vi "MartinsDCtemp.vi"() -> ()   [LabVIEW 2011]
uses:
  Sub VIs/Trap cluster.ctl
  <vilib>/Utility/inputDevices.llb/closeKeyboard.vi
  <vilib>/Utility/inputDevices.llb/keyboardAcquire.vi
  <vilib>/Utility/file.llb/Write To Spreadsheet File (DBL).vi
  <vilib>/vision/driver/NI_Vision_Acquisition_Software.lvlib
panel:
  in  "e_desired":sgl=0.5
  in  "Apply Corrections":bool
  in  "View Licence":bool
  in  "ok":bool caption="Mark the center of \nthe spot using the \nzoom and the point\ntool, then click this \nbutton"
  in  "Stop program":bool
  in  "Updating trap cluster":bool
  out "Camera enabled":bool
  out "SLM enabled":bool
  in  "Run calibration":bool
  in  "Hologram generation":cluster{"Method":i32, "Iterations":i32}={"Method"=0, "Iterations"=10} {"Method" items=["Lenses & Gratings (3D)", " Gerchberg-Saxton (3D)", "Gerchberg-Saxton FFT (2D)"]}
  in  "Display hologram\nand computed \nimage plane":bool=TRUE
  in  "ROI":T1={"Global Rectangle"=[309, 286, 371, 364], "Contours"=[{"Contour Type"=0, "ROI Type"=1, "Points"=[370, 286]}, {"Contour Type"=0, "ROI Type"=1, "Points"=[351, 363]}, {"Contour Type"=0, "ROI Type"=1, "Points"=[309, 315]}]}
  out "Image":T2(plugin-control)
  in  "Filename":string="test"
  out "appended path":path
  in  "File Path":path=path "C:/Users/Martin/Dropbox/GU/CUDA/GenerateHologramCUDA/LabVIEW/MartinDC/Measurements"
  in  "Save images":bool
  in  "Show image":bool=TRUE
  in  "ROI size":dbl=2.0 min=2.0 step=2.0
  in  "#images":i32=10
  in  "Tab Control":enum32{"Normal", "Grid"}(tab)=enum."Grid"
  in  "Z":dbl[](array[numeric])=[0.0, 0.0, 0.0]
  in  "I":dbl[](array[numeric])=[10.0, 10.0, 10.0]
  out "#":i32[](array[numeric])=[0, 1, 2]
  in  "G":bool[](array[boolean])=[FALSE, FALSE, FALSE]
  in  "Spots y":i32=3
  in  "Grid spacing":i32=32
  in  "Spots x":i32=3
  out "Calculated image plane":dbl[][](graph)
  out "Current trap pos":T3
  out "NI Vision error":errorcluster
  out "CUDA/SLM error":errorcluster
  in  "Cancel calibration":bool
  in  "Skip step if \ntimed out":bool
  in  "Display path":bool=TRUE
  out "Average step time (ms)":dbl
  in  "Step time \n(ms)":u32=10
  in  "Pause":bool
  in  "cancel path":bool
  out "Step skipped":bool
  in  "Path controls":T4={"follow path"=FALSE, "Step length"=1.0, "Arrive \nsimultaneously"=TRUE, "Synchronize traps"=FALSE, "Add current \npositions to path"=FALSE}
  in  "Create path":bool
  in  "Positioning  mode":enum16{"Normal", "Group", "Grid"}(ring)=enum."Grid"
  in  "Move \nHandle":bool
  out "Displayed Hologram":u8[][](graph)
  in  "Coordinate mapping \n(IMAQ to SLM)":T5={"sX"=-256.0, "sY"=-256.0, "sZ"=0.0, "cX"=0.5, "cY"=0.5, "cZ"=1.0}
  in  "Switch X/Y":bool
  # "Martin\nPersson 2011"
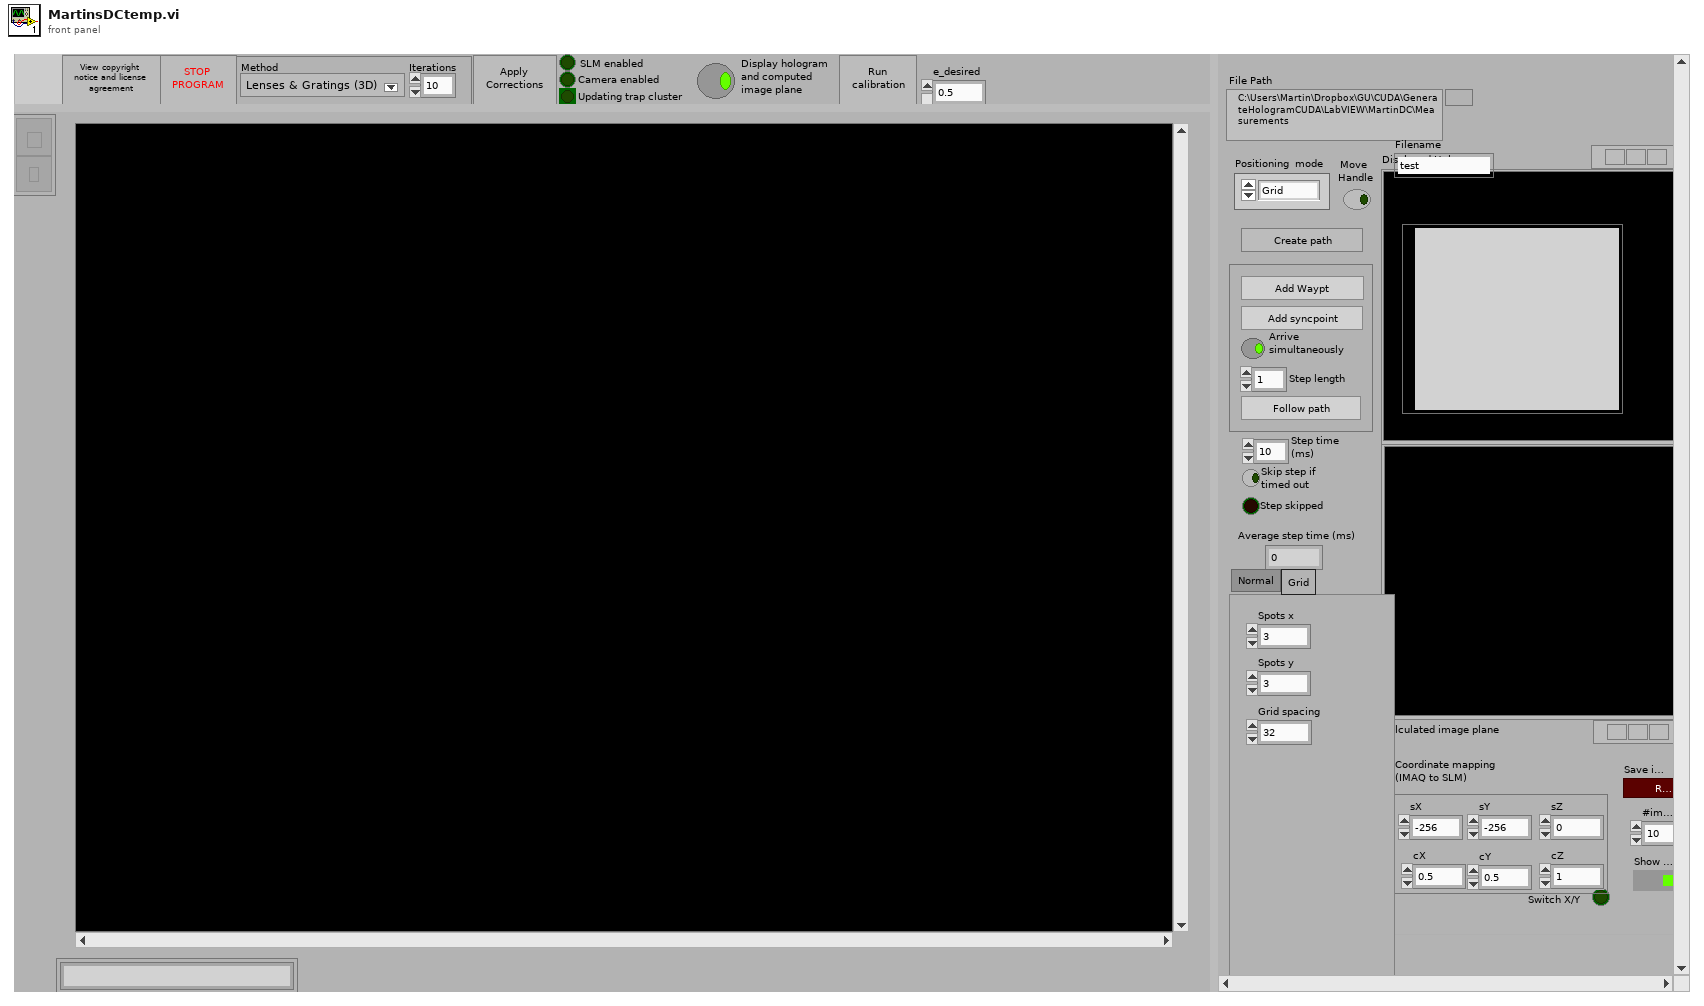
[diagram p1: front panel]
types:
  T1 = cluster{"Global Rectangle":i32[], "Contours":cluster{"Contour Type":u32, "ROI Type":u32, "Points":i32[]}[]}
  T2 = typedef "IMAQ Image.ctl" = refnum<image>
  T3 = typedef "Trap cluster.ctl" = cluster{"X (IMAQ)":dbl[], "Y (IMAQ)":dbl[], "Z":dbl[], "Amplitudes":dbl[], "Trap number":i32[], "ROI number":i32[], "Number of traps":i32, "Group":bool[]}
  T4 = cluster{"follow path":bool, "Step length":dbl, "Arrive \nsimultaneously":bool, "Synchronize traps":bool, "Add current \npositions to path":bool}
  T5 = cluster{"sX":dbl, "sY":dbl, "sZ":dbl, "cX":dbl, "cY":dbl, "cZ":dbl}
  T6 = cluster{"Centroid X":dbl[], "Centroid Y":dbl[], "Acquired Buffer Number":u32}
  T7 = typedef "IMAQdx.ctl" = refnum<k21>
  T8 = typedef "Image Type" = u32
  T9 = enum16{"0", "1", "2", "3", "4", "5", "6", "7", "8", "9", "A", "B", "C", "D", "E", "F", "G", "H", "I", "J", "K", "L", "M", "N", "O", "P", "Q", "R", "S", "T", "U", "V", "W", "X", "Y", "Z", "F1", "F2", "F3", "F4", "F5", "F6", "F7", "F8", "F9", "F10", "F11", "F12", "F13", "F14", "F15", "ADD", "BACK", "BACKSLASH", "CAPITAL", "COMMA", "DECIMAL", "DELETE", "DIVIDE", "DOWN", "END", "EQUALS", "ESCAPE", "GRAVE (`)", "HOME", "INSERT", "LBRACKET", "LCONTROL", "LEFT", "L ALT", "LSHIFT", "LWIN", "MINUS", "MULTIPLY", "NEXT", "NUMLOCK", "NUMPAD_0", "NUMPAD_1", "NUMPAD_2", "NUMPAD_3", "NUMPAD_4", "NUMPAD_5", "NUMPAD_6", "NUMPAD_7", "NUMPAD_8", "NUMPAD_9", "PAUSE", "PERIOD", "PRIOR (PG UP)", "RBRACKET", "RCONTROL", "RETURN", "RIGHT", "R ALT", "RSHIFT", "RWIN", "SCROLL", "SEMICOLON", "SLASH", "SPACE", "SUBTRACT", "TAB", "UP", "ENTER (num pad)", "' (quote)"}[]
  T10 = typedef "LVRectTypeDef.ctl" = cluster{"left":i16, "top":i16, "right":i16, "bottom":i16}
  T11 = cluster{"Contour Type":u32, "ROI Type":u32, "Points":i32[]}[]
  T12 = cluster{"Contour Type":u32, "ROI Type":u32, "Points":i32[]}
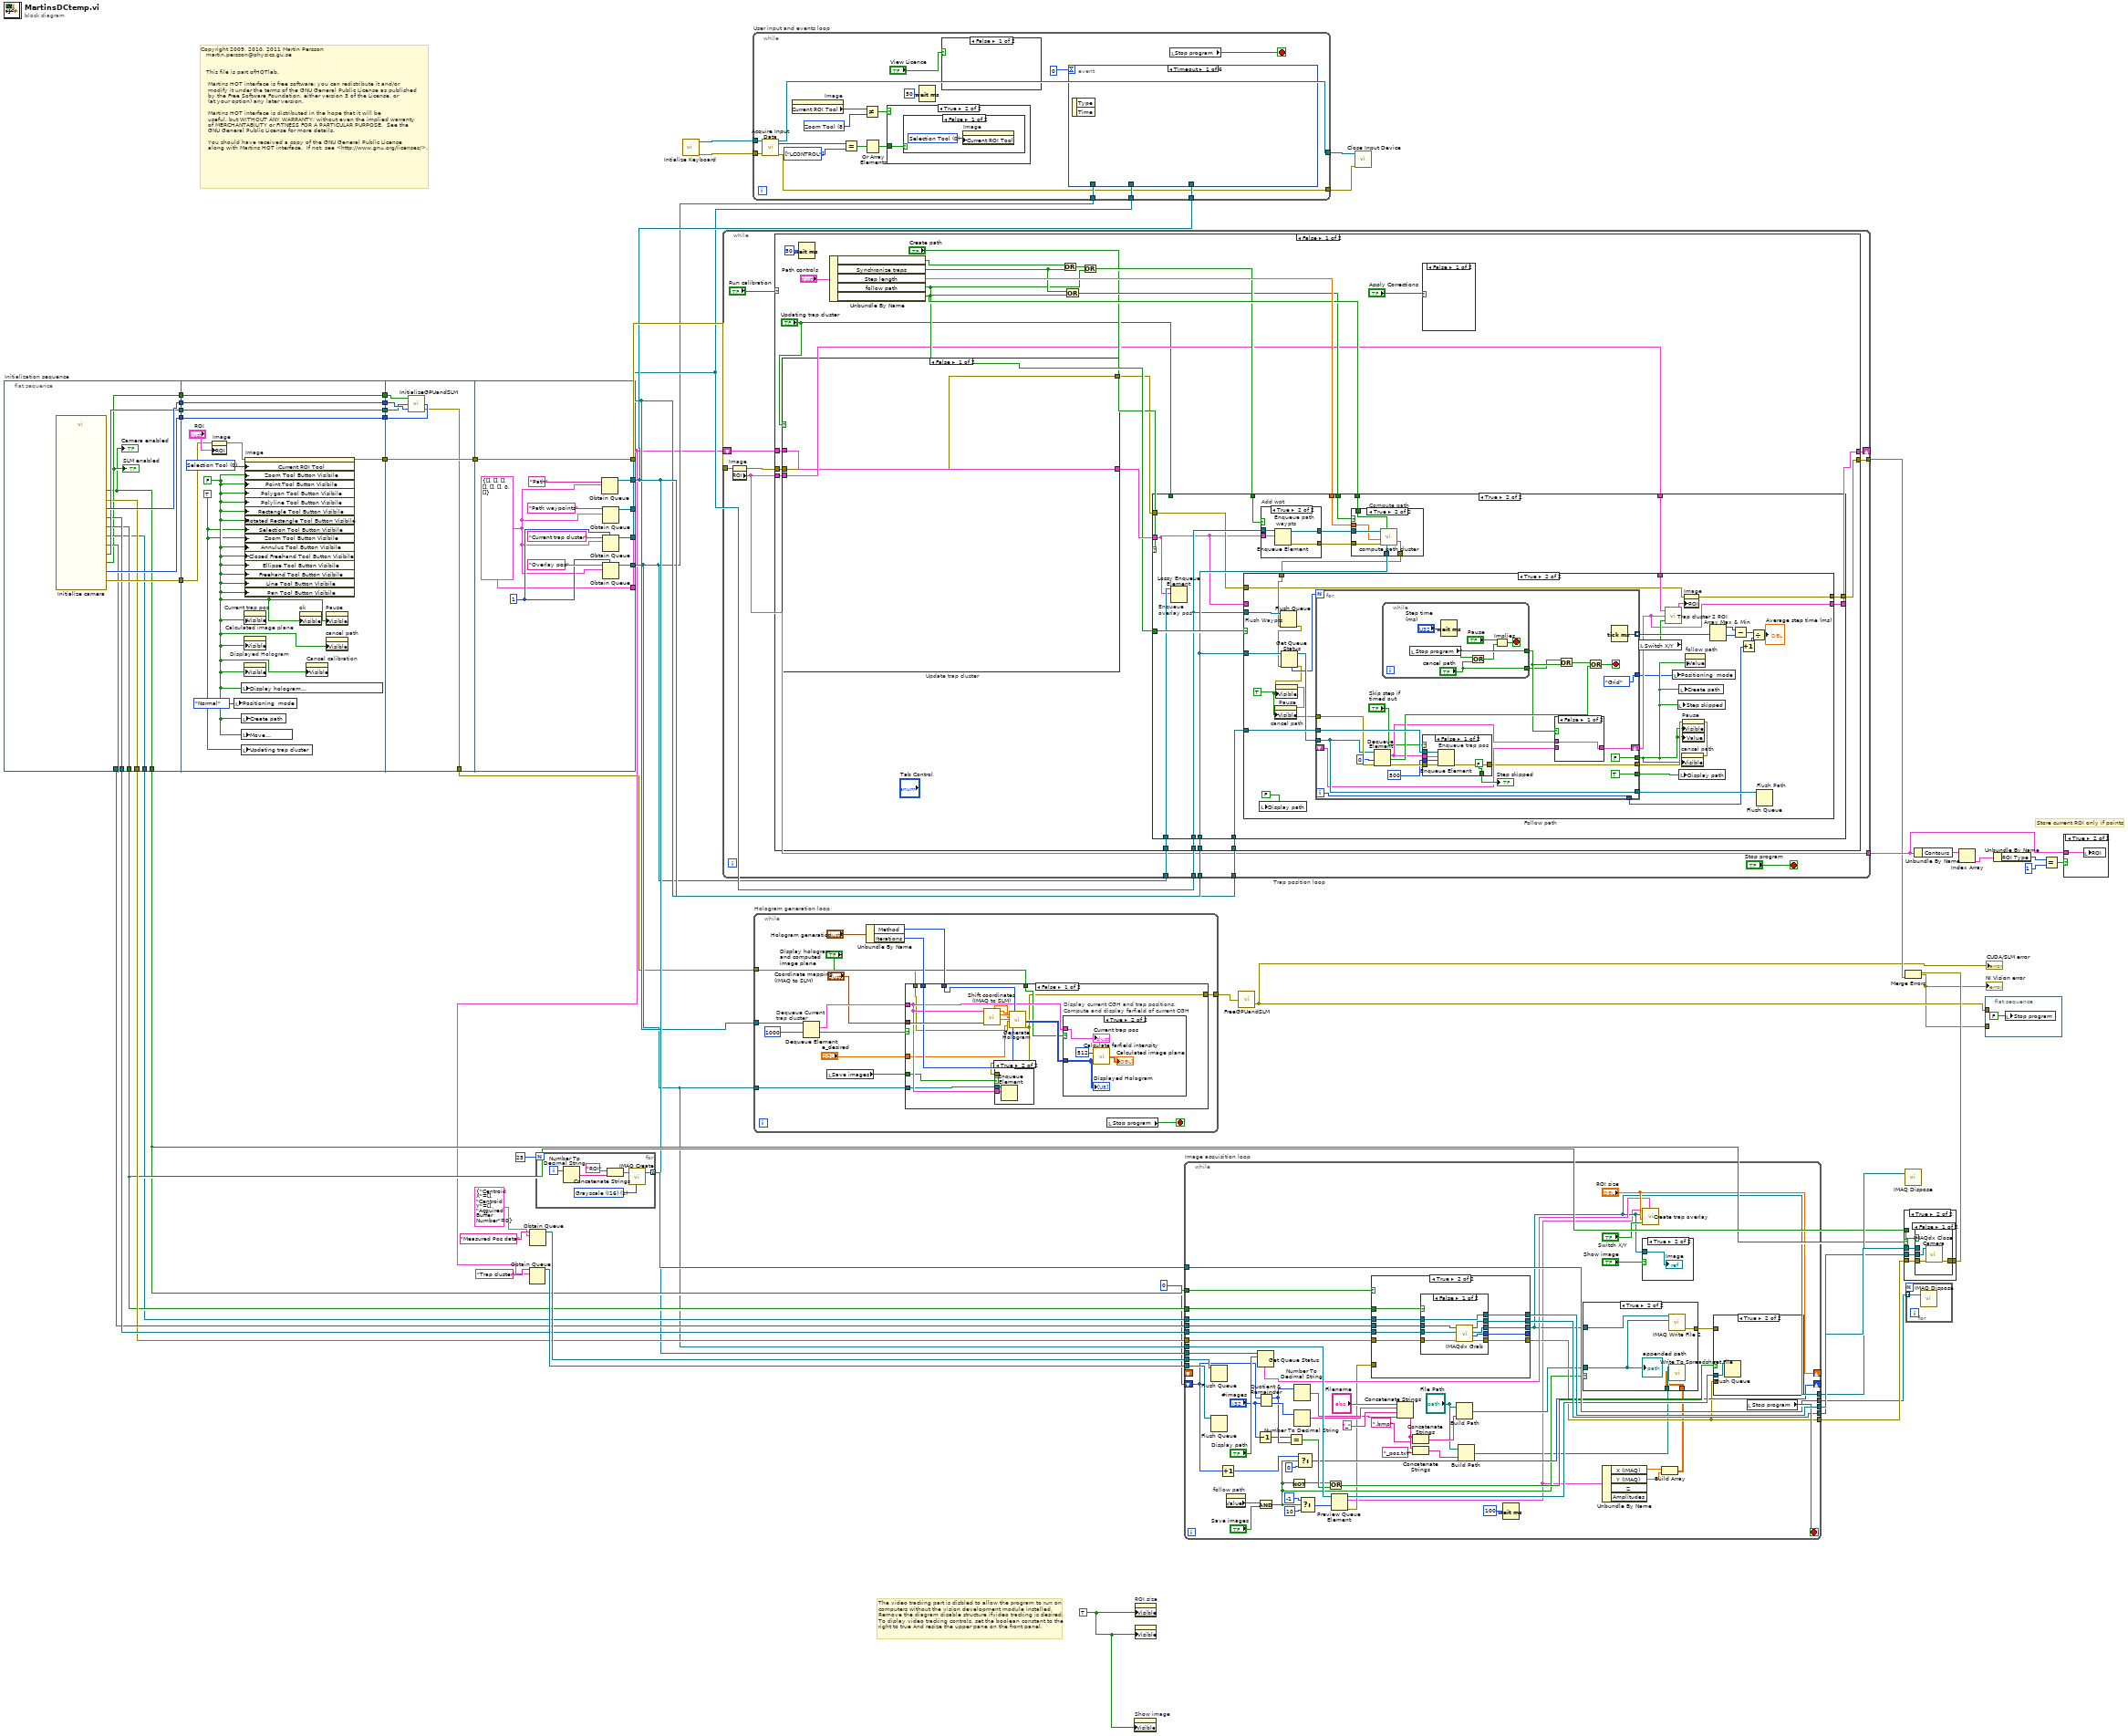
[diagram p0: block diagram]
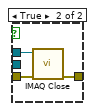
[diagram p3: hidden frame]
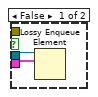
[diagram p4: hidden frame]
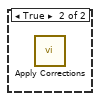
[diagram p7: hidden frame]
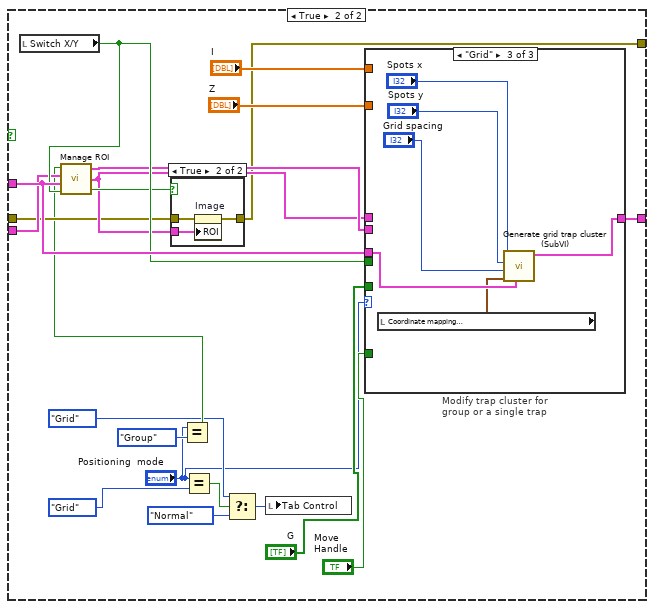
[diagram p8: hidden frame]
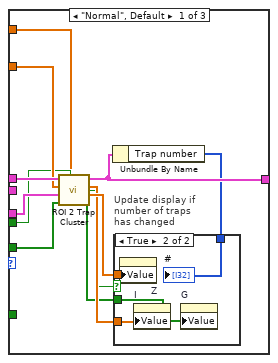
[diagram p10: hidden frame]
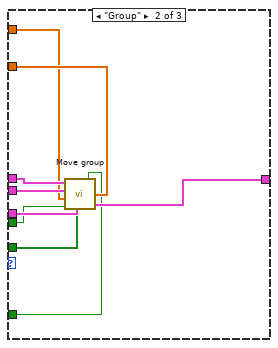
[diagram p12: hidden frame]
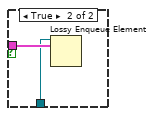
[diagram p14: hidden frame]
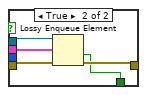
[diagram p16: hidden frame]
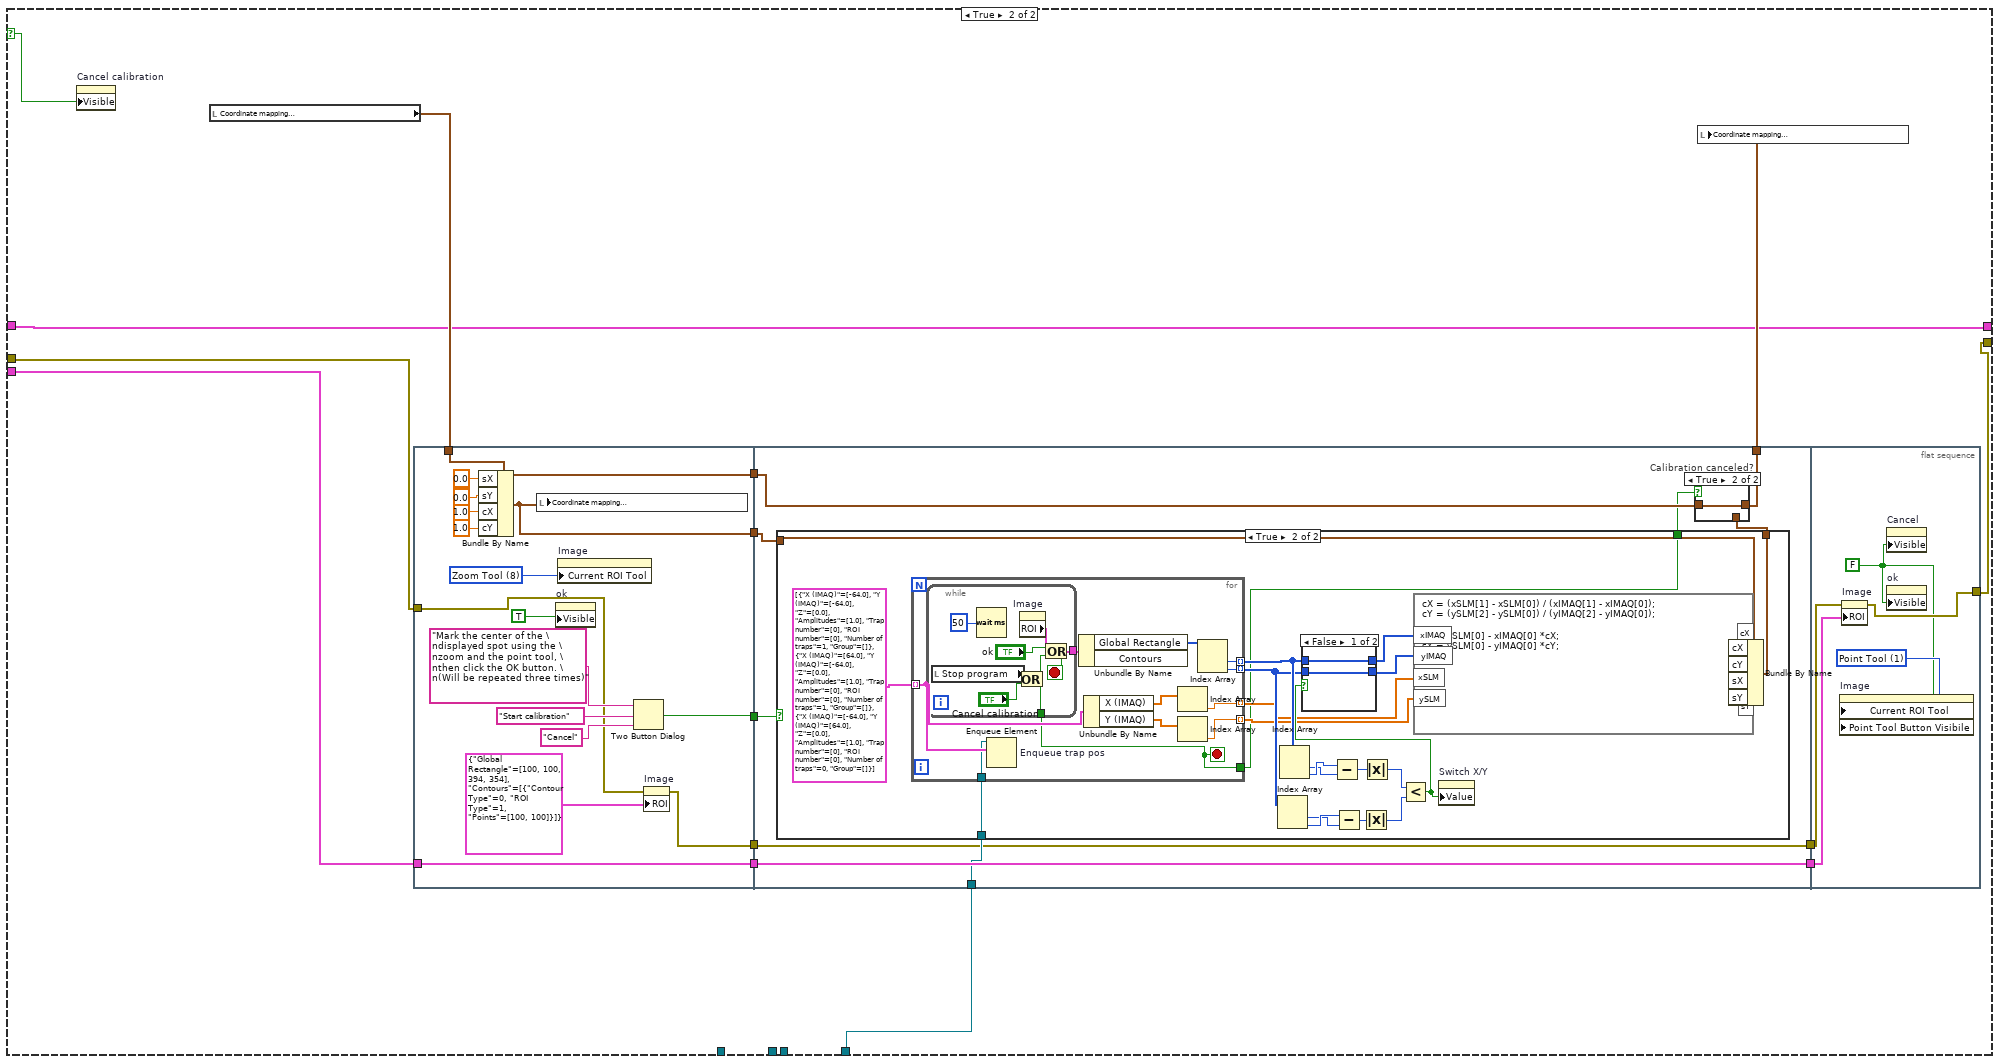
[diagram p20: hidden frame]
diagram:
  w40 = TRUE ("Visible")
  # "Copyright 2009, 2010, 2011 Martin Persson \n   martin.persson@physics.gu.se\n\n\n   This file is part ofHOTlab.\n\n    Martins HOT interface is free software: you can redistribute it and/or \n    modify it under the terms of the GNU General Public License as published \n    by the Free Software Foundation, either version 3 of the License, or\n    (at your option) any later version.\n\n    Martins HOT interface is distributed in the hope that it will be \n    useful, but WITHOUT ANY WARRANTY; without even the implied warranty\n    of MERCHANTABILITY or FITNESS FOR A PARTICULAR PURPOSE.  See the\n    GNU General Public License for more details.\n\n    You should have received a copy of the GNU General Public License\n    along with Martins HOT interface.  If not, see <http://www.gnu.org/licenses/>."
  # "Store current ROI only if points"
  # "The video tracking part is disbled to allow the program to run on\ncomputers without the vision development module installed. \nRemove the diagram disable structure ifvideo tracking is desired. \nTo diplay video tracking controls, set the boolean constant to the \nright to true And resize the upper pane on the front panel."
  n1 = flat-sequence "Initialization sequence" {
    tunnel: [w55] -> w25
    tunnel: [w64] -> w24
    tunnel: [w63] -> w23
    tunnel: [w62] -> w22
    tunnel: [w61] -> w21
    tunnel: [w60] -> w19
    tunnel: [w59] -> w18
    tunnel: [w58] -> w17
    tunnel: [w57] -> w16
    tunnel: [w56] -> w15
    tunnel: [w54] -> w14
    tunnel: w25 -> [w73]
    tunnel: w24 -> [w71]
    tunnel: w23 -> [w76]
    tunnel: w22 -> [w75]
    tunnel: w21 -> [w74]
    tunnel: [w73] -> w8
    tunnel: [w66] -> w7
    tunnel: [w76] -> w5
    tunnel: [w75] -> w4
    tunnel: [w74] -> w3
    tunnel: w8 -> [w79]
    tunnel: w7 -> [w82]
    tunnel: [w82] -> w6
    tunnel: w5 -> [w80]
    tunnel: w4 -> [w81]
    tunnel: w3 -> [w78]
    tunnel: [w77] -> w2
    tunnel: [w93] -> w20
    tunnel: w6 -> [w93]
    tunnel: [w91] -> w13
    tunnel: [w89] -> w12
    tunnel: [w87] -> w11
    tunnel: [w86] -> w10
    tunnel: [w83] -> w9
    frame #0 {
      n2 = call "Initialize camera.vi"() -> ("CUDA device ID"=w62:i32, "IMAQdx Session Out"=w59:T7, "TrueFrame out"=w63:i32, "IMAQ camera"=w57:bool, "Image reference out"=w60:T2, "SLM enabled"=w55:bool, "Camera enabled"=w54:bool, "Vision error out"=w64:errorcluster, "LUT path out"=w61:path, "IMAQ Session Out"=w56:refnum<k11>, "Camera error"=w58:errorcluster)  [unwired: 5 in]
      "Camera enabled" <- w54
      "SLM enabled" <- w55
    }
    frame #1 {
      w69 = TRUE ("ROI Tool Buttons Visibile:Zoom Tool Button Visible")
      w70 = FALSE ("ROI Tool Buttons Visibile:Zoom Tool Button Visible")
      w68 = u32 0 items=["Zoom Tool"=8, "Selection Tool"=0, "Pan Tool"=9, "Point Tool"=1, "Line Tool"=2, "Rectangle Tool"=3, "Rotated Rectangle Tool"=12, "Polyline Tool"=10, "Polygon Tool"=5, "Freehand Tool"=11, "Closed Freehand Tool"=6, "Ellipse Tool"=4, "Annulus Tool"=7] ("Current ROI Tool")
      n3 = property on="Image" class="ImageControl"(error in=w71, "ROI"="ROI") -> (error out=w67:errorcluster)  [unwired: 1 in, 1 out]
      n4 = local write "Positioning  mode"(enum16{"Normal", "Group", "Grid"}."Normal" ("Positioning  mode")) -> ()
      n5 = local write "Display hologram\nand computed \nimage plane"(w70) -> ()
      n6 = local write "Create path"(w70) -> ()
      n7 = local write "Move \nHandle"(w70) -> ()
      n8 = local write "Updating trap cluster"(w69) -> ()
      n9 = property on="Current trap pos" class="Clust (strict)"("Visible"=w70) -> ()  [unwired: 2 in, 2 out]
      n10 = property on="Calculated image plane" class="IntGraph (strict)"("Visible"=w70) -> ()  [unwired: 2 in, 2 out]
      n11 = property on="Displayed Hologram" class="IntGraph (strict)"("Visible"=w70) -> ()  [unwired: 2 in, 2 out]
      n12 = property on="Image" class="ImageControl"(error in=w67, "Current ROI Tool"=w68, "Zoom Tool Button Visibile"=w70, "Point Tool Button Visibile"=w70, "Polygon Tool Button Visibile"=w70, "Polyline Tool Button Visibile"=w70, "Rectangle Tool Button Visibile"=w70, "Rotated Rectangle Tool Button Visibile"=w70, "Selection Tool Button Visibile"=w69, "Zoom Tool Button Visibile"=w69, "Annulus Tool Button Visibile"=w70, "Closed Freehand Tool Button Visibile"=w70, "Ellipse Tool Button Visibile"=w70, "Freehand Tool Button Visibile"=w70, "Line Tool Button Visibile"=w70, "Pan Tool Button Visibile"=w70) -> (error out=w66:errorcluster)  [unwired: 1 in, 1 out]
      n13 = property on="ok" class="Bool"("Visible"=w70) -> ()  [unwired: 2 in, 2 out]
      n14 = property on="Cancel calibration" class="Bool"("Visible"=w70) -> ()  [unwired: 2 in, 2 out]
      n15 = property on="Pause" class="Bool (strict)"("Visible"=w70) -> ()  [unwired: 2 in, 2 out]
      n16 = property on="cancel path" class="Bool"("Visible"=w70) -> ()  [unwired: 2 in, 2 out]
    }
    frame #2 {
      n17 = call "InitializeGPUandSLM.vi"("TrueFrame"=w80, "deviceId"=w81, "Path to LUT file"=w78, "SLM enabled"=w79) -> ("CUDA/SLM error"=w77:errorcluster)  [unwired: 1 out]
    }
    frame #3 {
      w84 = 1 ("max queue size (-1, unlimited)")
      w83 = T3 {"X (IMAQ)"=[], "Y (IMAQ)"=[], "Z"=[], "Amplitudes"=[], "Trap number"=[], "ROI number"=[], "Number of traps"=0, "Group"=[]} ("output cluster 2")
      n18 = Obtain Queue(name (unnamed)="Path", element data type=w83) -> (queue out=w91:refnum<queue>)  [unwired: 3 in, 2 out]
      n19 = Obtain Queue(name (unnamed)="Path waypoints", element data type=w83) -> (queue out=w89:refnum<queue>)  [unwired: 3 in, 2 out]
      n20 = Obtain Queue(max queue size (-1, unlimited)=w84, name (unnamed)="Current trap cluster", element data type=w83) -> (queue out=w87:refnum<queue>)  [unwired: 2 in, 2 out]
      n21 = Obtain Queue(max queue size (-1, unlimited)=w84, name (unnamed)="Overlay pos", element data type=w83) -> (queue out=w86:refnum<queue>)  [unwired: 2 in, 2 out]
    }
  }
  n22 = Obtain Queue(name (unnamed)="Trap cluster", element data type=w9) -> (queue out=w45:refnum<queue>)  [unwired: 3 in, 2 out]
  n23 = Obtain Queue(name (unnamed)="Measured Pos data", element data type=T6 {"Centroid X"=[], "Centroid Y"=[], "Acquired Buffer Number"=0} ("output cluster 2")) -> (queue out=w48:refnum<queue>)  [unwired: 3 in, 2 out]
  n24 = for {
    N: 25 -> [_]
    tunnel: [w99] -> w50 mode=indexing
    i -> [w95]
    w97 = T8 1 items=["Grayscale (U8)", "Grayscale (I16)", "Grayscale (SGL)", "Complex (CSG)", "RGB (U32)", "HSL (U32)", "RGB (U64)", "Grayscale (U16)"] ("Image Type")
    n25 = Number To Decimal String(number=w95) -> (decimal integer string=w94:string)  [unwired: 1 in]
    n26 = Concatenate Strings("ROI" ("Image Name"), w94) -> (w96:string)
    n27 = call "IMAQ Create"("Image Name"=w96, "Image Type"=w97) -> ("New Image"=w99:T2)  [unwired: 3 in, 1 out]
  }
  n28 = call <vilib>:"Intialize Keyboard.vi"() -> ("error out"=w27:errorcluster, "device ID"=w53:refnum<k1>)  [unwired: 1 in, 9 out]
  n29 = while "Trap position loop" {
    tunnel: w12 -> [w111]
    tunnel: w13 -> [w108]
    shift-right: [w110] -> _
    shift-left: w9 -> [w103]
    tunnel: w11 -> [w109]
    tunnel: w10 -> [w106]
    tunnel: [w105] -> w34
    tunnel: w20 -> [w102]
    tunnel: [w100] -> w32
    stop <- "Stop program" stop-if-true
    n30 = property on="Image" class="ImageControl"(error in=w102) -> (error out=w101:errorcluster, "ROI"=w105:T1)  [unwired: 1 in, 1 out]
    n31 = case shown="False" "Run calibration" {
      selector: "Run calibration" -> [_ w304]
      tunnel: w111 -> [w135 _]
      tunnel: w103 -> [w134 w303]
      tunnel: [w113 w303] -> w110
      tunnel: w109 -> [w124 w313]
      tunnel: w108 -> [w122 _]
      tunnel: w106 -> [w119 _]
      tunnel: w105 -> [w118 w312]
      tunnel: w101 -> [w117 w308]
      tunnel: [w115 w305] -> w100
      frame False {
        n32 = case "Update trap cluster" shown="False" "Updating trap cluster" {
          tunnel: w134 -> [w137 w158]
          tunnel: [w137 w151] -> w125
          tunnel: w118 -> [_ w149]
          tunnel: w117 -> [w136 w148]
          tunnel: [w136 w147] -> w116
          frame False {
          }
          frame True {
            n33 = local read "Switch X/Y"() -> (w157:bool)
            n34 = Equal?(x="Positioning  mode", y=enum16{"Normal", "Group", "Grid"}."Group") -> (x = y?=w145:bool)
            n35 = call "Manage ROI.vi"("Switch X/Y"=w157, "Trap cluster in"=w158, "ROI in"=w149, "Group traps"=w145) -> ("Replace ROI"=w156:bool, "ROI out"=w150:T1, "Previous ROI out"=w155:T1)
            n36 = case shown="True" w156 {
              tunnel: w150 -> [_ w162]
              tunnel: w148 -> [w159 w161]
              tunnel: [w159 w160] -> w147
              frame False {
              }
              frame True {
                n37 = property on="Image" class="ImageControl"(error in=w161, "ROI"=w162) -> (error out=w160:errorcluster)  [unwired: 1 in, 1 out]
              }
            }
            n38 = Equal?(x="Positioning  mode", y=enum16{"Normal", "Group", "Grid"}."Grid") -> (x = y?=w143:bool)
            n39 = Select(t=enum32{"Normal", "Grid"}."Grid", s=w143, f=enum32{"Normal", "Grid"}."Normal" ("Tab Control")) -> (s? t:f=w140:enum32{"Normal", "Grid"})
            n40 = local write "Tab Control"(w140) -> ()
            n41 = case "Modify trap cluster for \ngroup or a single trap" shown="\"Grid\"" "Positioning  mode" {
              tunnel: [w167 w184 w189] -> w151
              tunnel: w150 -> [w174 w185 _]
              tunnel: w158 -> [w173 w187 w190]
              tunnel: w155 -> [_ w186 _]
              tunnel: "Z" -> [w172 w183 _]
              tunnel: "Move \nHandle" -> [_ w182 _]
              tunnel: w157 -> [w171 w181 _]
              tunnel: "I" -> [w169 w180 _]
              tunnel: "G" -> [w164 w179 _]
              frame "Normal", Default {
                n42 = call "ROI 2 Trap Cluster.vi"("Amplitudes"=w169, "Switch X/Y"=w171, "Group"=w164, "Trap Cluster in"=w173, "Z"=w172, "ROI"=w174) -> ("Group out"=w163:bool[], "Z out"=w170:dbl[], "Amplitudes out"=w168:dbl[], "Trap Cluster Out"=w167:T3, "Update display"=w165:bool)
                n43 = Unbundle By Name(w167) -> ("Trap number"=w166:i32[])
                n44 = case "Update display if\nnumber of traps \nhas changed" shown="True" w165 {
                  tunnel: w170 -> [_ w178]
                  tunnel: w168 -> [_ w177]
                  tunnel: w166 -> [_ w176]
                  tunnel: w163 -> [_ w175]
                  frame False {
                  }
                  frame True {
                    n45 = property on="Z" class="Arr (strict)"("Value"=w178) -> ()  [unwired: 2 in, 2 out]
                    n46 = property on="I" class="Arr (strict)"("Value"=w177) -> ()  [unwired: 2 in, 2 out]
                    n47 = property on="G" class="Arr (strict)"("Value"=w175) -> ()  [unwired: 2 in, 2 out]
                    "#" <- w176
                  }
                }
              }
              frame "Group" {
                n48 = call "Move group.vi"("New handle position in"=w185, "Trap cluster in"=w187, "Previous handle position in"=w186, "Amplitudes"=w180, "Group"=w179, "Switch X/Y"=w181, "Move handle"=w182, "Z"=w183) -> ("Trap cluster out"=w184:T3)
              }
              frame "Grid" {
                n49 = local read "Coordinate mapping \n(IMAQ to SLM)"() -> (w188:T5)
                n50 = call "Generate grid trap cluster (SubVI).vi"("output cluster 3"=w190, "Coordinate mapping \n(IMAQ to SLM)"=w188, "Grid spacing"="Grid spacing", "Spots y"="Spots y", "Spots x"="Spots x") -> ("output cluster 2"=w189:T3)  [unwired: 6 in]
              }
            }
          }
        }
        n51 = Wait (ms)(milliseconds to wait=u32 50) -> ()  [unwired: 1 out]
        n52 = Unbundle By Name("Path controls") -> ("Add current \npositions to path"=w120:bool, "Synchronize traps"=w129:bool, "Step length"=w132:dbl, "follow path"=w123:bool, "Arrive \nsimultaneously"=w131:bool)
        n53 = Or(x=w120, y=w129) -> (x .or. y?=w130:bool)
        n54 = Or(x=w129, y=w123) -> (x .or. y?=w127:bool)
        n55 = Or(x=w130, y=w123) -> (x .or. y?=w128:bool)
        n56 = case shown="True" "Create path" {
          tunnel: w135 -> [_ w206]
          tunnel: w125 -> [w194 w200]
          tunnel: w132 -> [_ w215]
          tunnel: w122 -> [_ w210]
          tunnel: w131 -> [_ w214]
          tunnel: w128 -> [_ w213]
          tunnel: w127 -> [_ w212]
          tunnel: w123 -> [_ w211]
          tunnel: w124 -> [w197 w207]
          tunnel: w119 -> [_ w205]
          tunnel: w118 -> [_ w204]
          tunnel: w116 -> [w196 w203]
          tunnel: [w196 w202] -> w115
          tunnel: "Updating trap cluster" -> [w195 _]
          tunnel: [w194 w201] -> w113
          frame False {
            n57 = case shown="False" w195 {
              tunnel: w194 -> [_ w199]
              tunnel: w197 -> [_ w198]
              frame False {
              }
              frame True {
                n58 = Lossy Enqueue Element(queue=w198, element=w199) -> ()  [unwired: 1 in, 4 out]
              }
            }
          }
          frame True {
            n59 = Lossy Enqueue Element "Enqueue\noverlay pos"(queue=w205, element=w200) -> ()  [unwired: 1 in, 4 out]
            n60 = case "Add wpt" shown="True" w213 {
              tunnel: w200 -> [_ w294]
              tunnel: w206 -> [w291 w295]
              tunnel: [w291 w292] -> w216
              tunnel: [_ w293] -> w208
              frame False {
              }
              frame True {
                n61 = Enqueue Element "Enqueue path\n waypts"(queue=w295, element=w294) -> (queue out=w292:refnum<queue>, error out=w293:errorcluster)  [unwired: 2 in, 1 out]
              }
            }
            n62 = case "Compute path" shown="True" w212 {
              tunnel: w216 -> [_ w302]
              tunnel: w210 -> [_ w301]
              tunnel: w215 -> [_ w300]
              tunnel: w214 -> [_ w299]
              tunnel: [w296 w297] -> w209
              tunnel: w208 -> [w296 w298]
              frame False {
              }
              frame True {
                n63 = call "compute path cluster.vi"("path queue"=w301, "Arrive simultaeously"=w299, "error in (no error)"=w298, "Step length\n(IMAQ pixels)"=w300, "waypoint queue"=w302) -> ("error out"=w297:errorcluster)  [unwired: 2 in]
              }
            }
            n64 = case "Follow path" shown="True" w211 {
              tunnel: w210 -> [_ w246]
              tunnel: w209 -> [_ w247]
              tunnel: w207 -> [_ w249]
              tunnel: w206 -> [_ w248]
              tunnel: w204 -> [_ w245]
              tunnel: w203 -> [w218 w226]
              tunnel: [w218 w225] -> w202
              tunnel: [w217 w220] -> w201
              tunnel: w200 -> [w217 _]
              frame False {
              }
              frame True {
                w240 = TRUE ("Visible")
                n65 = local write "Display path"(FALSE ("Display path")) -> ()
                n66 = Flush Queue "Flush Waypts"(queue=w248, error in (no error)=w247) -> (error out=w239:errorcluster)  [unwired: 2 out]
                n67 = Get Queue Status(queue=w246, error in (no error)=w239) -> (queue out=w243:refnum<queue>, error out=w238:errorcluster, # elements in queue=w242:i32)  [unwired: 1 in, 5 out]
                n68 = property on="Pause" class="Bool (strict)"(error in=w238, "Visible"=w240) -> (error out=w237:errorcluster)  [unwired: 1 in, 1 out]
                n69 = property on="cancel path" class="Bool"(error in=w237, "Visible"=w240) -> (error out=w236:errorcluster)  [unwired: 1 in, 1 out]
                n70 = for {
                  N: w242 -> [_]
                  tunnel: w236 -> [w269]
                  tunnel: w249 -> [w271]
                  tunnel: w243 -> [w267]
                  tunnel: [w267] -> w241
                  tunnel: [FALSE ("Group traps")] -> w221
                  shift-right: [w258] -> w220
                  shift-left: _ -> [w260]
                  tunnel: [w257] -> w235
                  tunnel: [w254] -> w233 mode=indexing
                  tunnel: [w255] -> w229
                  tunnel: [TRUE ("Display path")] -> w227
                  tunnel: [enum16{"Normal", "Group", "Grid"}."Grid" ("Positioning  mode")] -> w219
                  i -> [w255]
                  stop <- w264 stop-if-true
                  n71 = Dequeue Element(queue=w267, timeout in ms (-1)=0, error in (no error)=w269) -> (element=w259:T3, timed out?=w263:bool, error out=w270:errorcluster)  [unwired: 1 out]
                  n72 = while {
                    tunnel: [w288] -> w261
                    tunnel: ["cancel path"] -> w256
                    stop <- w290 stop-if-true
                    n73 = local read "Stop program"() -> (w288:bool)
                    n74 = Wait (ms)(milliseconds to wait="Step time \n(ms)") -> ()  [unwired: 1 out]
                    n75 = Or(x=w288, y="cancel path") -> (x .or. y?=w286:bool)
                    n76 = Implies(1:w286, 2:"Pause") -> (0:w290:bool)
                  }
                  n77 = case shown="False" "Skip step if \ntimed out" {
                    tunnel: w271 -> [w277 w282]
                    tunnel: w270 -> [w276 w280]
                    tunnel: [FALSE ("overflow?") w278] -> w262
                    tunnel: w259 -> [w275 w281]
                    tunnel: [w274 w279] -> w257
                    tunnel: 500 ("timeout in ms (-1)") -> [w273 _]
                    frame False {
                      n78 = Enqueue Element "Enqueue trap pos"(queue=w277, element=w275, timeout in ms (-1)=w273, error in (no error)=w276) -> (error out=w274:errorcluster)  [unwired: 2 out]
                    }
                    frame True {
                      n79 = Lossy Enqueue Element(queue=w282, element=w281, error in (no error)=w280) -> (overflow?=w278:bool, error out=w279:errorcluster)  [unwired: 2 out]
                    }
                  }
                  "Step skipped" <- w262
                  n80 = case shown="False" w261 {
                    tunnel: w260 -> [_ w284]
                    tunnel: w259 -> [w283 _]
                    tunnel: [w283 w284] -> w258
                    frame False {
                    }
                    frame True {
                    }
                  }
                  n81 = Or(x=w256, y=w261) -> (x .or. y?=w266:bool)
                  n82 = Or(x=w266, y=w263) -> (x .or. y?=w264:bool)
                  n83 = Tick Count (ms)() -> (millisecond timer value=w254:u32)
                }
                n84 = local read "Switch X/Y"() -> (w223:bool)
                n85 = call "Trap cluster 2 ROI.vi"("Switch X/Y"=w223, "Trap cluster"=w220, "ROI in"=w245) -> ("ROI out"=w244:T1)
                n86 = local write "Positioning  mode"(w219) -> ()
                n87 = local write "Step skipped"(w221) -> ()
                n88 = local write "Display path"(w227) -> ()
                n89 = local write "Create path"(w221) -> ()
                n90 = property on="Pause" class="Bool (strict)"(error in=w235, "Visible"=w221, "Value"=w221) -> (error out=w234:errorcluster)  [unwired: 1 in, 1 out]
                n91 = property on="cancel path" class="Bool"(error in=w234, "Visible"=w221) -> ()  [unwired: 1 in, 2 out]
                n92 = property on="Image" class="ImageControl"(error in=w226, "ROI"=w244) -> (error out=w225:errorcluster)  [unwired: 1 in, 1 out]
                n93 = property on="follow path" class="Bool (strict)"("Value"=w221) -> ()  [unwired: 2 in, 2 out]
                n94 = Array Max & Min(array=w233) -> (max value=w232:u32, min value=w231:u32)  [unwired: 2 out]
                n95 = Subtract(x=w232, y=w231) -> (x-y=w230:u32)
                n96 = Increment(x=w229) -> (x+1=w224:i32)
                n97 = Divide(x=w230, y=w224) -> (x/y=→"Average step time (ms)":dbl)
                n98 = Flush Queue "Flush Path"(queue=w241) -> ()  [unwired: 1 in, 3 out]
              }
            }
          }
        }
        n99 = case shown="False" "Apply Corrections" {
          frame False {
          }
          frame True {
            n100 = call "Apply Corrections.vi"() -> ()  [unwired: 1 in]
          }
        }
      }
      frame True {
        n101 = property on="Cancel calibration" class="Bool"("Visible"=w304) -> ()  [unwired: 2 in, 2 out]
        n102 = local read "Coordinate mapping \n(IMAQ to SLM)"() -> (w311:T5)
        n103 = flat-sequence {
          tunnel: [w327] -> w317
          tunnel: [w329] -> w316
          tunnel: w312 -> [w327]
          tunnel: w311 -> [w321]
          tunnel: [w318] -> w310
          tunnel: [w321] -> w309
          tunnel: w308 -> [w320]
          tunnel: [w319] -> w306
          tunnel: [w342] -> w315
          tunnel: w317 -> [w342]
          tunnel: w316 -> [w336]
          tunnel: [w338] -> w314
          tunnel: w313 -> [w341]
          tunnel: w310 -> [w340]
          tunnel: w309 -> [w337]
          tunnel: [w334] -> w307
          tunnel: w306 -> [w334]
          tunnel: w315 -> [w397]
          tunnel: w307 -> [w395]
          tunnel: [w394] -> w305
          frame #0 {
            w330 = u32 8 items=["Zoom Tool"=8, "Selection Tool"=0, "Pan Tool"=9, "Point Tool"=1, "Line Tool"=2, "Rectangle Tool"=3, "Rotated Rectangle Tool"=12, "Polyline Tool"=10, "Polygon Tool"=5, "Freehand Tool"=11, "Closed Freehand Tool"=6, "Ellipse Tool"=4, "Annulus Tool"=7] ("Current ROI Tool")
            n104 = Bundle By Name(cluster=w321, "sX"=0.0, "sY"=0.0, "cX"=1.0 ("sX"), "cY"=1.0) -> (w318:T5)
            n105 = local write "Coordinate mapping \n(IMAQ to SLM)"(w318) -> ()
            n106 = property on="ok" class="Bool"("Visible"=TRUE ("ROI Tool Buttons Visibile:Zoom Tool Button Visible")) -> ()  [unwired: 2 in, 2 out]
            n107 = property on="Image" class="ImageControl"("Current ROI Tool"=w330) -> ()  [unwired: 2 in, 2 out]
            n108 = Two Button Dialog(message="Mark the center of the \ndisplayed spot using the \nzoom and the point tool, \nthen click the OK button. \n(Will be repeated three times)", 1:"Cancel" ("F button name (\"Cancel\")"), 2:"Start calibration" ("T button name (\"OK\")")) -> (T button?=w329:bool)
            n109 = property on="Image" class="ImageControl"(error in=w320, "ROI"=T1 {"Global Rectangle"=[100, 100, 394, 354], "Contours"=[{"Contour Type"=0, "ROI Type"=1, "Points"=[100, 100]}]} ("ROI 2")) -> (error out=w319:errorcluster)  [unwired: 1 in, 1 out]
          }
          frame #1 {
            n110 = case shown="True" w336 {
              tunnel: w340 -> [w346 w357]
              tunnel: [w346 w352] -> w339
              tunnel: w341 -> [_ w348]
              tunnel: [TRUE ("Stop program") w347] -> w335
              frame False {
              }
              frame True {
                n111 = for {
                  tunnel: [w384] -> w366 mode=indexing
                  tunnel: [w383] -> w365 mode=indexing
                  tunnel: T3[] [{"X (IMAQ)"=[-64.0], "Y (IMAQ)"=[-64.0], "Z"=[0.0], "Amplitudes"=[1.0], "Trap number"=[0], "ROI number"=[0], "Number of traps"=1, "Group"=[]}, {"X (IMAQ)"=[64.0], "Y (IMAQ)"=[-64.0], "Z"=[0.0], "Amplitudes"=[1.0], "Trap number"=[0], "ROI number"=[0], "Number of traps"=1, "Group"=[]}, {"X (IMAQ)"=[-64.0], "Y (IMAQ)"=[64.0], "Z"=[0.0], "Amplitudes"=[1.0], "Trap number"=[0], "ROI number"=[0], "Number of traps"=0, "Group"=[]}] -> [w381] mode=indexing
                  tunnel: [w378] -> w350 mode=indexing
                  tunnel: [w376] -> w349 mode=indexing
                  tunnel: w348 -> [w380]
                  tunnel: [w375] -> w347
                  stop <- w375 stop-if-true
                  n112 = while {
                    tunnel: [w391] -> w382
                    tunnel: [w387] -> w375
                    stop <- w389 stop-if-true
                    n113 = local read "Stop program"() -> (w388:bool)
                    n114 = Wait (ms)(milliseconds to wait=u32 50) -> ()  [unwired: 1 out]
                    n115 = Or(x=w388, y="Cancel calibration") -> (x .or. y?=w387:bool)
                    n116 = property on="Image" class="ImageControl"() -> ("ROI"=w391:T1)  [unwired: 2 in, 2 out]
                    n117 = Or(x="ok", y=w387) -> (x .or. y?=w389:bool)
                  }
                  n118 = Enqueue Element "Enqueue trap pos"(queue=w380, element=w381) -> ()  [unwired: 2 in, 3 out]
                  n119 = Unbundle By Name(w382) -> ("Global Rectangle"=w385:i32[])  [unwired: 1 out]
                  n120 = Unbundle By Name(w381) -> ("X (IMAQ)"=w379:dbl[], "Y (IMAQ)"=w377:dbl[])
                  n121 = Index Array(array=w379) -> (element=w378:dbl)  [unwired: 1 in]
                  n122 = Index Array(array=w377) -> (element=w376:dbl)  [unwired: 1 in]
                  n123 = Index Array(array=w385) -> (element #1=w384:i32, element #2=w383:i32)  [unwired: 2 in]
                }
                n124 = Index Array(array=w365) -> (element #1=w367:i32, element #2=w368:i32)  [unwired: 2 in]
                n125 = Index Array(array=w366) -> (element #1=w369:i32, element #2=w370:i32)  [unwired: 2 in]
                n126 = Subtract(x=w370, y=w369) -> (x-y=w362:i32)
                n127 = Subtract(x=w368, y=w367) -> (x-y=w360:i32)
                n128 = Absolute Value(x=w360) -> (abs(x)=w359:i32)
                n129 = Absolute Value(x=w362) -> (abs(x)=w361:i32)
                n130 = Less?(x=w361, y=w359) -> (x < y?=w358:bool)
                n131 = case shown="False" w358 {
                  tunnel: w366 -> [w372 w374]
                  tunnel: w365 -> [w371 w373]
                  tunnel: [w371 w374] -> w363
                  tunnel: [w372 w373] -> w364
                  frame False {
                  }
                  frame True {
                  }
                }
                n132 = formula code="cX = (xSLM[1] - xSLM[0]) / (xIMAQ[1] - xIMAQ[0]); \ncY = (ySLM[2] - ySLM[0]) / (yIMAQ[2] - yIMAQ[0]); \n\nsX = xSLM[0] - xIMAQ[0] *cX;\nsY = ySLM[0] - yIMAQ[0] *cY;"("xIMAQ"=w364, "yIMAQ"=w363, "xSLM"=w350, "ySLM"=w349) -> ("cX"=w356:dbl, "cY"=w355:dbl, "sX"=w354:dbl, "sY"=w353:dbl)
                n133 = property on="Switch X/Y" class="Bool (strict)"("Value"=w358) -> ()  [unwired: 2 in, 2 out]
                n134 = Bundle By Name(cluster=w357, "cX"=w356, "cY"=w355, "sX"=w354, "sY"=w353) -> (w352:T5)
              }
            }
            n135 = case "Calibration canceled?" shown="True" w335 {
              tunnel: w339 -> [w343 _]
              tunnel: [w343 w344] -> w338
              tunnel: w337 -> [_ w344]
              frame False {
              }
              frame True {
              }
            }
          }
          frame #2 {
            w393 = FALSE ("ROI Tool Buttons Visibile:Zoom Tool Button Visible")
            w396 = u32 1 items=["Zoom Tool"=8, "Selection Tool"=0, "Pan Tool"=9, "Point Tool"=1, "Line Tool"=2, "Rectangle Tool"=3, "Rotated Rectangle Tool"=12, "Polyline Tool"=10, "Polygon Tool"=5, "Freehand Tool"=11, "Closed Freehand Tool"=6, "Ellipse Tool"=4, "Annulus Tool"=7] ("Current ROI Tool")
            n136 = property on="Image" class="ImageControl"("Current ROI Tool"=w396, "Point Tool Button Visibile"=w393) -> ()  [unwired: 2 in, 2 out]
            n137 = property on="Image" class="ImageControl"(error in=w395, "ROI"=w397) -> (error out=w394:errorcluster)  [unwired: 1 in, 1 out]
            n138 = property on="Cancel" class="Bool"("Visible"=w393) -> ()  [unwired: 2 in, 2 out]
            n139 = property on="ok" class="Bool"("Visible"=w393) -> ()  [unwired: 2 in, 2 out]
          }
        }
        n140 = local write "Coordinate mapping \n(IMAQ to SLM)"(w314) -> ()
      }
    }
  }
  n141 = while "User input and events loop" {
    tunnel: w53 -> [w415]
    tunnel: w10 -> [w404]
    tunnel: w12 -> [w403]
    tunnel: w13 -> [w402]
    tunnel: [w401] -> w28
    tunnel: w27 -> [w400]
    tunnel: [w399] -> w26
    stop <- w407 stop-if-true
    w412 = u32 8 items=["Zoom Tool"=8, "Selection Tool"=0, "Pan Tool"=9, "Point Tool"=1, "Line Tool"=2, "Rectangle Tool"=3, "Rotated Rectangle Tool"=12, "Polyline Tool"=10, "Polygon Tool"=5, "Freehand Tool"=11, "Closed Freehand Tool"=6, "Ellipse Tool"=4, "Annulus Tool"=7] ("Current ROI Tool")
    w409 = T9 [enum."LCONTROL"] items=["0", "1", "2", "3", "4", "5", "6", "7", "8", "9", "A", "B", "C", "D", "E", "F", "G", "H", "I", "J", "K", "L", "M", "N", "O", "P", "Q", "R", "S", "T", "U", "V", "W", "X", "Y", "Z", "F1", "F2", "F3", "F4", "F5", "F6", "F7", "F8", "F9", "F10", "F11", "F12", "F13", "F14", "F15", "ADD", "BACK", "BACKSLASH", "CAPITAL", "COMMA", "DECIMAL", "DELETE", "DIVIDE", "DOWN", "END", "EQUALS", "ESCAPE", "GRAVE (`)", "HOME", "INSERT", "LBRACKET", "LCONTROL", "LEFT", "L ALT", "LSHIFT", "LWIN", "MINUS", "MULTIPLY", "NEXT", "NUMLOCK", "NUMPAD_0", "NUMPAD_1", "NUMPAD_2", "NUMPAD_3", "NUMPAD_4", "NUMPAD_5", "NUMPAD_6", "NUMPAD_7", "NUMPAD_8", "NUMPAD_9", "PAUSE", "PERIOD", "PRIOR (PG UP)", "RBRACKET", "RCONTROL", "RETURN", "RIGHT", "R ALT", "RSHIFT", "RWIN", "SCROLL", "SEMICOLON", "SLASH", "SPACE", "SUBTRACT", "TAB", "UP", "ENTER (num pad)", "' (quote)"] ("keys pressed")
    n142 = call-poly <vilib>:"Acquire Input Data.vi"("device ID"=w415, "error in (no error)"=w400) -> ("device ID"=w401:refnum<k1>, "keys pressed"=w408:T9, "error out"=w399:errorcluster)  [unwired: 15 out]
    n143 = property on="Image" class="ImageControl"() -> ("Current ROI Tool"=w411:u32)  [unwired: 2 in, 2 out]
    n144 = Equal?(x=w408, y=w409) -> (x = y?=w410:bool[])
    n145 = Not Equal?(x=w411, y=w412) -> (x != y?=w413:bool)
    n146 = Or Array Elements(Boolean array=w410) -> (logical OR=w414:bool)
    n147 = case shown="True" w413 {
      tunnel: w414 -> [_ w436]
      frame False {
      }
      frame True {
        n148 = case shown="False" w436 {
          frame False {
            w437 = u32 0 items=["Zoom Tool"=8, "Selection Tool"=0, "Pan Tool"=9, "Point Tool"=1, "Line Tool"=2, "Rectangle Tool"=3, "Rotated Rectangle Tool"=12, "Polyline Tool"=10, "Polygon Tool"=5, "Freehand Tool"=11, "Closed Freehand Tool"=6, "Ellipse Tool"=4, "Annulus Tool"=7] ("Current ROI Tool")
            n149 = property on="Image" class="ImageControl"("Current ROI Tool"=w437) -> ()  [unwired: 2 in, 2 out]
          }
          frame True {
            w438 = u32 1 items=["Zoom Tool"=8, "Selection Tool"=0, "Pan Tool"=9, "Point Tool"=1, "Line Tool"=2, "Rectangle Tool"=3, "Rotated Rectangle Tool"=12, "Polyline Tool"=10, "Polygon Tool"=5, "Freehand Tool"=11, "Closed Freehand Tool"=6, "Ellipse Tool"=4, "Annulus Tool"=7] ("Current ROI Tool")
            n150 = property on="Image" class="ImageControl"("Current ROI Tool"=w438) -> ()  [unwired: 2 in, 2 out]
          }
        }
      }
    }
    n151 = Wait (ms)(milliseconds to wait=u32 50) -> ()  [unwired: 1 out]
    n152 = case shown="False" "View Licence" {
      frame False {
      }
      frame True {
        n153 = call "View license.vi"() -> ()  [unwired: 1 in]
      }
    }
    n154 = event shown="[0] Timeout" {
      selector: _ -> [_ _ _ _ _ _]
      dyn-events: _ -> [_ _ _ _ _ _]
      timeout: 0 -> [_ _ _ _ _ _]
      tunnel: w404 -> [_ _ w426 _ _ _]
      tunnel: w403 -> [_ _ w425 _ _ _]
      tunnel: w402 -> [_ _ w429 _ _ _]
      event Timeout {
        n155 = event-data() -> ()  [unwired: 1 in, 2 out]
      }
      event "Display hologram\nand computed \nimage plane": Value Change {
        n156 = event-data() -> ("NewVal"=w417:bool)  [unwired: 1 in, 4 out]
        n157 = property on="Current trap pos" class="Clust (strict)"("Visible"=w417) -> ()  [unwired: 2 in, 2 out]
        n158 = property on="Displayed Hologram" class="IntGraph (strict)"("Visible"=w417) -> ()  [unwired: 2 in, 2 out]
        n159 = property on="Calculated image plane" class="IntGraph (strict)"("Visible"=w417) -> ()  [unwired: 2 in, 2 out]
        n160 = property on="Property Node" class="VI"() -> ("Front Panel.WinBounds"=w424:T10)  [unwired: 2 in, 2 out]
        n161 = Unbundle By Name(w424) -> ("right"=w423:i16, "left"=w422:i16)
        n162 = Subtract(x=w423, y=w422) -> (x-y=w421:i16)
        n163 = Select(t=i16 500 ("x-y"), s=w417, f=i16 196 ("x-y")) -> (s? t:f=w416:i16)
        n164 = Subtract(x=w421, y=w416) -> (x-y=w420:i16)
        n165 = property on="Splitter" class="Splitter"("Position"=w420) -> ()  [unwired: 2 in, 2 out]
      }
      event "Create path": Value Change {
        n166 = event-data() -> ()  [unwired: 1 in, 5 out]
        n167 = property on="follow path" class="Bool (strict)"("Value"=FALSE) -> ()  [unwired: 2 in, 2 out]
        n168 = Flush Queue "Flush path \nwaypt queue"(queue=w425) -> ()  [unwired: 1 in, 3 out]
        n169 = Preview Queue Element(queue=w426) -> (element=w427:T3, error out=w430:errorcluster)  [unwired: 2 in, 2 out]
        n170 = Flush Queue "Flush path queue"(queue=w429) -> (queue out=w428:refnum<queue>)  [unwired: 1 in, 2 out]
        n171 = Enqueue Element "Enqueue current \ntrap pos in path"(queue=w428, element=w427) -> ()  [unwired: 2 in, 3 out]
        n172 = Enqueue Element "Enqueue current \ntrap pos in path \nwaypts"(queue=w425, element=w427, error in (no error)=w430) -> ()  [unwired: 1 in, 3 out]
      }
      event "cancel path": Value Change {
        n173 = event-data() -> ()  [unwired: 1 in, 5 out]
        n174 = local write "Create path"(FALSE ("Visible")) -> ()
      }
      event "Image", "Positioning  mode", "Z", "I", "Coordinate mapping \n(IMAQ to SLM)": Mouse Down {
        n175 = event-data() -> ()  [unwired: 1 in, 7 out]
        n176 = local write "Updating trap cluster"(TRUE ("Update trap positions")) -> ()
      }
      event "Positioning  mode", "Z", "I", "Image", "Coordinate mapping \n(IMAQ to SLM)": Mouse Up {
        n177 = event-data() -> ()  [unwired: 1 in, 7 out]
        n178 = flat-sequence {
          frame #0 {
            n179 = Wait (ms)(milliseconds to wait=u32 100) -> ()  [unwired: 1 out]
          }
          frame #1 {
            n180 = local write "Updating trap cluster"(FALSE ("Update trap positions")) -> ()
          }
        }
      }
    }
    n181 = local read "Stop program"() -> (w407:bool)
  }
  n182 = while "Hologram generation loop" {
    tunnel: w11 -> [w449]
    tunnel: w10 -> [w439]
    tunnel: w2 -> [w443]
    tunnel: [w442] -> w31
    stop <- w450 stop-if-true
    n183 = Dequeue Element "Dequeue Current \ntrap cluster"(queue=w449, timeout in ms (-1)=1000) -> (element=w448:T3, timed out?=w447:bool)  [unwired: 1 in, 2 out]
    n184 = local read "Save images"() -> (w440:bool)
    n185 = Unbundle By Name("Hologram generation") -> ("Method"=w453:i32, "Iterations"=w452:i32)
    n186 = case shown="False" w447 {
      tunnel: "Coordinate mapping \n(IMAQ to SLM)" -> [w468 _]
      tunnel: "Display hologram\nand computed \nimage plane" -> [w458 _]
      tunnel: w453 -> [w462 _]
      tunnel: w452 -> [w461 _]
      tunnel: w448 -> [w460 _]
      tunnel: w439 -> [w459 _]
      tunnel: w443 -> [w457 w477]
      tunnel: [w454 w477] -> w442
      tunnel: "e_desired" -> [w456 _]
      tunnel: w440 -> [w455 _]
      frame False {
        n187 = call "Shift coordinates (IMAQ to SLM).vi"("Trap cluster"=w460, "Coordinate mapping \n(IMAQ to SLM)"=w468) -> ("X (SLM)"=w463:sgl[], "Y (SLM)"=w466:sgl[], "Intensities"=w464:sgl[], "Z (SLM)"=w465:sgl[])  [unwired: 1 in, 1 out]
        n188 = call "Generate Hologram.vi"("x"=w463, "y"=w466, "z"=w465, "spot_intensities"=w464, "CUDA/SLM error in"=w457, "e_desired"=w456, "N_iterations"=w461, "method"=w462) -> ("CGH out"=w467:u8[][], "CUDA/SLM error out"=w454:errorcluster)  [unwired: 16 in, 2 out]
        n189 = case shown="True" w455 {
          tunnel: w460 -> [w470 w472]
          tunnel: w459 -> [w469 w471]
          tunnel: w454 -> [_ _]
          frame False {
            n190 = Lossy Enqueue Element(queue=w469, element=w470) -> ()  [unwired: 1 in, 4 out]
          }
          frame True {
            n191 = Enqueue Element(queue=w471, element=w472) -> ()  [unwired: 2 in, 3 out]
          }
        }
        n192 = case "Display current CGH and trap positions.\nCompute and display farfield of current CGH" shown="True" w458 {
          tunnel: w467 -> [_ w475]
          tunnel: w460 -> [_ w474]
          frame False {
          }
          frame True {
            n193 = call "Calculate farfield intensity.vi"("h_pSLM"=w475, "Numeric"=512) -> ("Calculated image plane"=→"Calculated image plane":dbl[][])
            "Displayed Hologram" <- w475
            "Current trap pos" <- w474
          }
        }
      }
      frame True {
      }
    }
    n194 = local read "Stop program"() -> (w450:bool)
  }
  n195 = property on="Show image" class="Bool (strict)"("Visible"=w40) -> ()  [unwired: 2 in, 2 out]
  n196 = property on="ROI size" class="DigNum (strict)"("Visible"=w40) -> ()  [unwired: 2 in, 2 out]
  n197 = property on="Save images" class="Bool (strict)"("Visible"=w40) -> ()  [unwired: 2 in, 2 out]
  n198 = while "Image acquisition loop" {
    tunnel: w14 -> [w519]
    tunnel: w19 -> [w535]
    tunnel: w15 -> [w534]
    tunnel: [w533] -> w52
    tunnel: [w495] -> w51
    tunnel: w50 -> [w529]
    tunnel: w48 -> [w521]
    shift-right: ["ROI size"] -> _
    shift-left: _ -> [_]
    tunnel: w45 -> [w520]
    tunnel: [w529] -> w43
    tunnel: [w510] -> w42
    tunnel: [w528] -> w41
    tunnel: w18 -> [w527]
    tunnel: w16 -> [w526]
    tunnel: w10 -> [w525]
    tunnel: w13 -> [w524]
    tunnel: w17 -> [w522]
    shift-right: [w498] -> _
    shift-left: 0 ("timeout in ms (-1)") -> [w497]
    stop <- w532 stop-if-true
    n199 = Flush Queue(queue=w521) -> ()  [unwired: 1 in, 3 out]
    n200 = Flush Queue(queue=w520) -> ()  [unwired: 1 in, 3 out]
    n201 = Increment(x=w497) -> (x+1=w496:i32)
    n202 = property on="follow path" class="Bool (strict)"() -> ("Value"=w511:bool)  [unwired: 2 in, 2 out]
    n203 = Decrement(x="#images") -> (x-1=w501:i32)
    n204 = Get Queue Status(queue=w524, return elements? (F)="Display path") -> (elements=w516:T3[])  [unwired: 1 in, 7 out]
    n205 = Quotient & Remainder(x=w497, y="#images") -> (x-y*floor(x/y)=w506:i32, floor(x/y)=w509:i32)
    n206 = And(x=w511, y="Save images") -> (x .and. y?=w491:bool)
    n207 = Equal?(x=w501, y=w506) -> (x = y?=w513:bool)
    n208 = Not(x=w491) -> (.not. x?=w499:bool)
    n209 = Number To Decimal String(number=w506) -> (decimal integer string=w505:string)  [unwired: 1 in]
    n210 = Number To Decimal String(number=w509) -> (decimal integer string=w508:string)  [unwired: 1 in]
    n211 = Select(t=w496, s=w491, f=0) -> (s? t:f=w498:i32)
    n212 = Select(t=-1, s=w491, f=10) -> (s? t:f=w490:i32)
    n213 = Or(x=w499, y=w513) -> (x .or. y?=w500:bool)
    n214 = Preview Queue Element(queue=w525, timeout in ms (-1)=w490) -> (queue out=w512:refnum<queue>, element=w488:T3, error out=w489:errorcluster)  [unwired: 1 in, 1 out]
    n215 = case shown="True" w519 {
      tunnel: w535 -> [w544 w555]
      tunnel: w534 -> [w543 w554]
      tunnel: [w543 w553] -> w533
      tunnel: [w542 w552] -> w495
      tunnel: [w544 w551] -> w510
      tunnel: [w545 w550] -> w528
      tunnel: w527 -> [w545 w549]
      tunnel: w526 -> [_ w548]
      tunnel: w522 -> [w542 w547]
      tunnel: [_ w546] -> _
      tunnel: w489 -> [_ _]
      frame False {
      }
      frame True {
        n216 = case shown="False" w548 {
          tunnel: w555 -> [w563 w571]
          tunnel: [w561 w570] -> w553
          tunnel: [w560 w569] -> w552
          tunnel: w554 -> [w561 w568]
          tunnel: [w562 w567] -> w551
          tunnel: [w557 w566] -> w546
          tunnel: [w559 w565] -> w550
          tunnel: w549 -> [w558 w565]
          tunnel: w547 -> [w556 w564]
          frame False {
            n217 = call <vilib>:"IMAQdx Grab.vi"("error in"=w556, "Image In"=w563, "Session In"=w558) -> ("error out"=w560:errorcluster, "Buffer Number Out"=w557:u32, "Image Out"=w562:T2, "Session Out"=w559:T7)  [unwired: 5 in]
          }
          frame True {
            n218 = call <vilib>:"IMAQ Grab Acquire.vi"("error in (no error)"=w564, "Image In"=w571, "IMAQ Session In"=w568) -> ("error out"=w569:errorcluster, "Acquired Buffer Number"=w566:u32, "Image Out"=w567:T2, "IMAQ Session Out"=w570:refnum<k11>)  [unwired: 1 in, 4 out]
          }
        }
      }
    }
    n219 = Concatenate Strings("Filename", w508, "_" ("string"), w505) -> (w485:string)
    n220 = Concatenate Strings(w485, ".bmp" ("string")) -> (w483:string)
    n221 = Concatenate Strings(w485, "_pos.txt" ("string")) -> (w480:string)
    n222 = Build Path(base path="File Path", name or relative path=w483) -> (appended path=w504:path)
    n223 = Build Path(base path="File Path", name or relative path=w480) -> (appended path=w479:path)
    n224 = Wait (ms)(milliseconds to wait=u32 100) -> ()  [unwired: 1 out]
    n225 = Unbundle By Name(w488) -> ("X (IMAQ)"=w487:dbl[], "Y (IMAQ)"=w486:dbl[])  [unwired: 2 out]
    n226 = call "Create trap overlay.vi"("Current trap cluster"=w488, "Image in"=w510, "ROI size"="ROI size", "Switch X/Y"="Switch X/Y", "Path"=w516) -> ()  [unwired: 1 out]
    n227 = case shown="True" "Show image" {
      tunnel: w510 -> [_ w572]
      frame False {
      }
      frame True {
        "Image" <- w572
      }
    }
    n228 = Build Array(w487, w486) -> (w478:dbl[][])
    n229 = case shown="True" w491 {
      tunnel: w510 -> [_ w540]
      tunnel: w504 -> [_ w539]
      tunnel: [_ w538] -> w494
      tunnel: w479 -> [_ w537]
      tunnel: w478 -> [_ w536]
      frame False {
      }
      frame True {
        n230 = call-poly "IMAQ Write File 2"("File Path"=w539, "Image"=w540) -> ("error out"=w538:errorcluster)  [unwired: 8 in, 1 out]
        n231 = call-poly <vilib>:"Write To Spreadsheet File.vi"("2D data"=w536, "file path (dialog if empty)"=w537) -> ()  [unwired: 6 in, 1 out]
        "appended path" <- w539
      }
    }
    n232 = case shown="True" w500 {
      tunnel: w512 -> [_ w541]
      tunnel: w495 -> [_ _]
      tunnel: w494 -> [_ _]
      frame False {
      }
      frame True {
        n233 = Flush Queue(queue=w541) -> ()  [unwired: 1 in, 3 out]
      }
    }
    n234 = local read "Stop program"() -> (w532:bool)
  }
  n235 = call "FreeGPUandSLM.vi"("error in"=w31) -> ("error out"=w30:errorcluster)  [unwired: 1 out]
  "CUDA/SLM error" <- w30
  n236 = call-poly <vilib>:"Close Input Device.vi"("error in (no error)"=w26, "device ID"=w28) -> ()  [unwired: 9 out]
  n237 = case shown="True" w14 {
    tunnel: w52 -> [_ w578]
    tunnel: w51 -> [w573 w577]
    tunnel: w41 -> [_ w576]
    tunnel: w16 -> [_ w575]
    tunnel: [w573 w574] -> w33
    frame False {
    }
    frame True {
      n238 = case shown="False" w575 {
        tunnel: w578 -> [_ w584]
        tunnel: w577 -> [w581 w583]
        tunnel: [w580 w582] -> w574
        tunnel: w576 -> [w579 _]
        frame False {
          n239 = call <vilib>:"IMAQdx Close Camera.vi"("error in"=w581, "Session In"=w579) -> ("error out"=w580:errorcluster)  [unwired: 9 in]
        }
        frame True {
          n240 = call <vilib>:"IMAQ Close.vi"("error in (no error)"=w583, "IMAQ Session In"=w584) -> ("error out"=w582:errorcluster)  [unwired: 9 in]
        }
      }
    }
  }
  n241 = Merge Errors(w33, w32) -> (w29:errorcluster)
  "NI Vision error" <- w29
  n242 = call "IMAQ Dispose"("Image"=w42) -> ()  [unwired: 5 in, 1 out]
  n243 = for {
    tunnel: w43 -> [w585] mode=indexing
    n244 = call "IMAQ Dispose"("Image"=w585) -> ()  [unwired: 5 in, 1 out]
  }
  n245 = Unbundle By Name(w34) -> ("Contours"=w39:T11)
  n246 = Index Array(array=w39) -> (element=w38:T12)  [unwired: 1 in]
  n247 = flat-sequence {
    tunnel: w30 -> [_]
    tunnel: w29 -> [_]
    frame #0 {
      n248 = local write "Stop program"(FALSE ("Stop program")) -> ()
    }
  }
  n249 = Unbundle By Name(w38) -> ("ROI Type"=w37:u32)
  n250 = Equal?(x=w37, y=u32 1) -> (x = y?=w35:bool)
  n251 = case shown="True" w35 {
    tunnel: w34 -> [_ w587]
    frame False {
    }
    frame True {
      n252 = local write "ROI"(w587) -> ()
    }
  }
